vi "Error Query.vi"(8 "error in (no error)":errorcluster, 11 "VISA resource name":refnum<visa-resource-name>) -> (0 "error out":errorcluster, 1 "Error Message":string, 2 "Error Code":i32[](array[numeric]), 3 "VISA resource name out":refnum<visa-resource-name>)   [LabVIEW 2024, in "Detector SCPI.lvlib"]
doc: "Queries the instrument for any errors in the instrument's error queue. It will continue to read errors until all errors have been read from the instrument. Any errors will be returned in the <B>error out</B> control.\n\n<B>Note:</B>\nThis VI is called automatically by most driver VIs so it is not usually necessary to call this in an application."
uses:
  <instrlib>/Detector SCPI/Detector SCPI.lvlib
panel:
  # "EDIT: Note: The Error Query VI is included as a subVI in all driver VIs except low-level API VIs. If the instrument does not support error query, then remove the VI and remove subVI calls in each instrument driver VI that calls it."
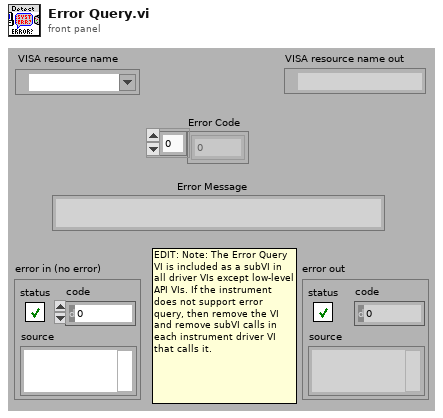
[diagram p1: front panel]
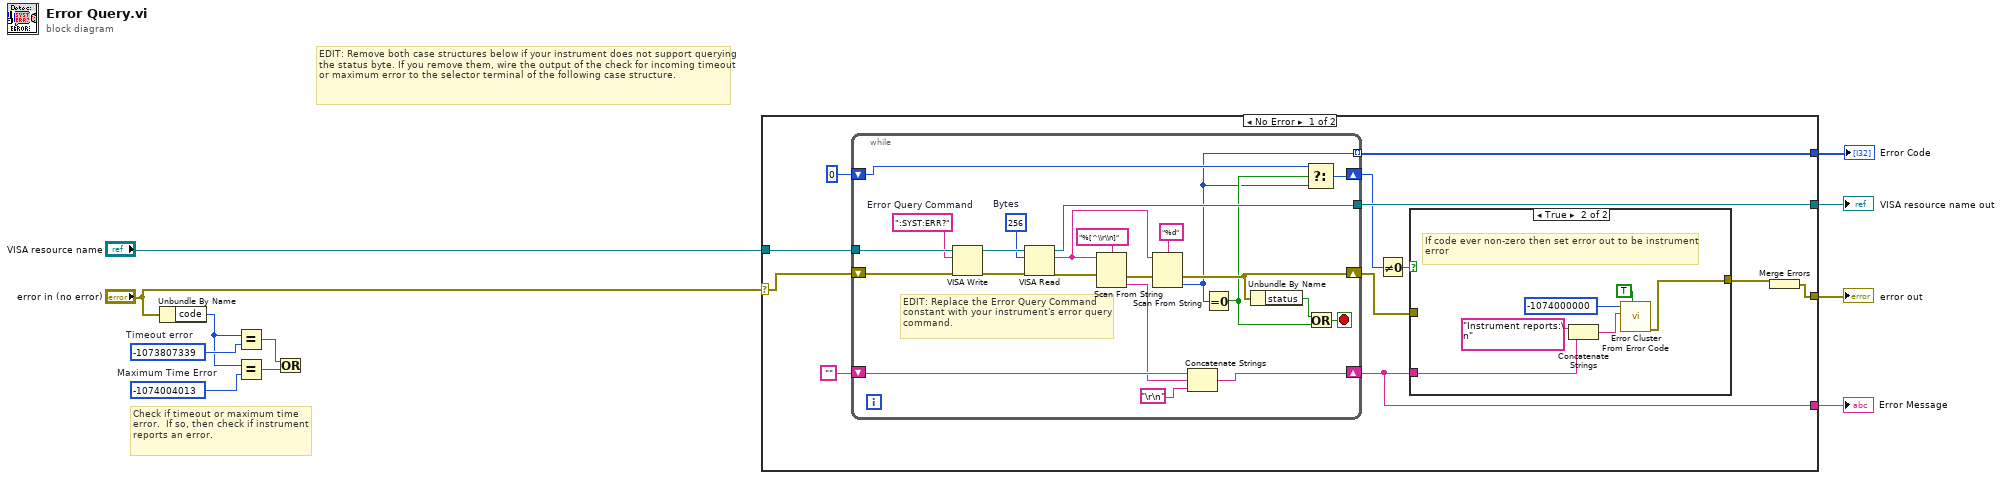
[diagram p0: block diagram]
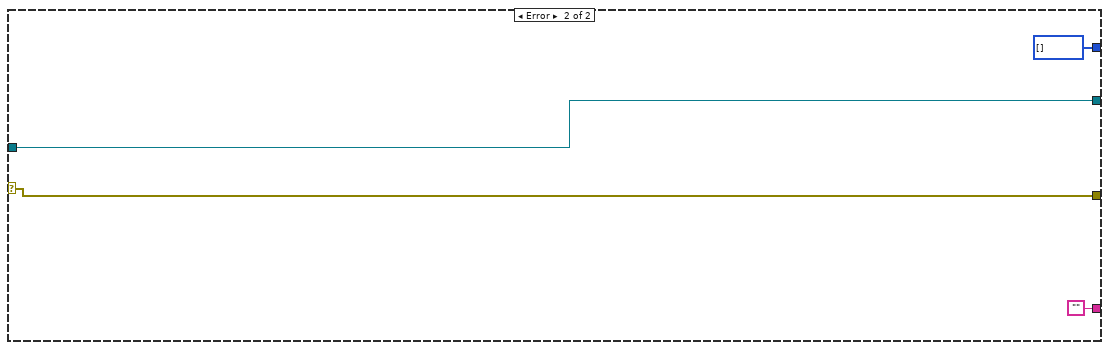
[diagram p3: hidden frame]
diagram:
  w4 = -1074004013  # Maximum Time Error
  w6 = -1073807339  # Timeout error
  # "Check if timeout or maximum time error.  If so, then check if instrument reports an error."
  # "EDIT: Remove both case structures below if your instrument does not support querying the status byte. If you remove them, wire the output of the check for incoming timeout or maximum error to the selector terminal of the following case structure."
  n1 = Unbundle By Name("error in (no error)") -> ("code"=w5:i32)
  n2 = Equal?(x=w5, y=w6) -> (x = y?=w2:bool)
  n3 = Equal?(x=w5, y=w4) -> (x = y?=w3:bool)
  n4 = Or(x=w2, y=w3) -> ()  [unwired: 1 out]
  n5 = case shown="No Error" "error in (no error)" {
    selector: "error in (no error)" -> [w12 w54]
    tunnel: [w23 w57] -> w11
    tunnel: "VISA resource name" -> [w22 w57]
    tunnel: [w20 w54] -> w10
    tunnel: [w15 ""] -> w9
    tunnel: [w14 i32[] []] -> w8
    frame No Error {
      n6 = while {
        tunnel: [w53] -> w23
        tunnel: w22 -> [w52]
        shift-right: [w40] -> w15
        shift-left: "" -> [w43]
        shift-right: [w38] -> w16
        shift-left: 0 -> [w39]
        shift-right: [w36] -> w13
        shift-left: w12 -> [w37]
        tunnel: [w31] -> w14 mode=indexing
        stop <- w46 stop-if-true
        w50 = u32 256  # Bytes
        w48 = ":SYST:ERR?"  # Error Query Command
        # "EDIT: Replace the Error Query Command constant with your instrument's error query command."
        n7 = VISA Write(VISA resource name=w52, write buffer=w48, error in (no error)=w37) -> (VISA resource name out=w51:refnum<visa-resource-name>, error out=w49:errorcluster)  [unwired: 1 out]
        n8 = VISA Read(VISA resource name=w51, byte count=w50, error in (no error)=w49) -> (VISA resource name out=w53:refnum<visa-resource-name>, read buffer=w44:string, error out=w35:errorcluster)  [unwired: 1 out]
        n9 = Scan From String(format string="%[^\\r\\n]", input string=w44, error in=w35) -> (error out=w34:errorcluster, output 1=w41:string)  [unwired: 2 in, 2 out]
        n10 = Scan From String(format string="%d", input string=w44, error in=w34) -> (error out=w36:errorcluster, output 1=w31:i32)  [unwired: 2 in, 2 out]
        n11 = Concatenate Strings(w43, w41, "\r\n") -> (w40:string)
        n12 = Equal To 0?(x=w31) -> (x = 0?=w32:bool)
        n13 = Unbundle By Name(w36) -> ("status"=w33:bool)
        n14 = Select(t=w39, s=w32, f=w31) -> (s? t:f=w38:i32)
        n15 = Or(x=w33, y=w32) -> (x .or. y?=w46:bool)
      }
      n16 = Not Equal To 0?(x=w16) -> (x != 0?=w18:bool)
      n17 = case shown="True" w18 {
        tunnel: w15 -> [_ w29]
        tunnel: [w24 w25] -> w17
        tunnel: w13 -> [w24 _]
        frame False {
        }
        frame True {
          # "If code ever non-zero then set error out to be instrument error"
          n18 = Concatenate Strings("Instrument reports:\n" ("Source"), w29) -> (w26:string)
          n19 = call <vilib>:"Error Cluster From Error Code.vi"("show call chain? (False)"=TRUE, "error message (\"\")"=w26, "error code (0)"=-1074000000 ("Code")) -> ("error out"=w25:errorcluster)  [unwired: 6 in]
        }
      }
      n20 = Merge Errors(w17) -> (w20:errorcluster)
    }
    frame Error {
    }
  }
  "VISA resource name out" <- w11
  "error out" <- w10
  "Error Message" <- w9
  "Error Code" <- w8
